vi "Deploy Host Interface.vi"(8 "error in":errorcluster caption="error in (no error)", 10 "resource":string) -> (0 "error out":errorcluster, 2 "resource out":string, 3 "lia host interface":refnum<class "LIA Host Interface.lvclass">)   [LabVIEW 2018, in "Lock-In Amplifier Example Shared.lvlib"]
uses:
  Lock-In Amplifier Example Shared.lvlib
  interface/Interface/LIA Host Interface.lvclass
  interface/Interface RT/LIA Host Interface RT.lvclass
  C:/Users/jfernand/Repositories/Lock-In-Amplifier/Shared/lib/interface/Interface/LIA Host Interface.lvclass
  interface/Interface FPGA/LIA Host Interface FPGA.lvclass
  <vilib>/nisyscfg/nisyscfg.lvlib
  <resource>/objmgr/niflexrioatomicsae.rc
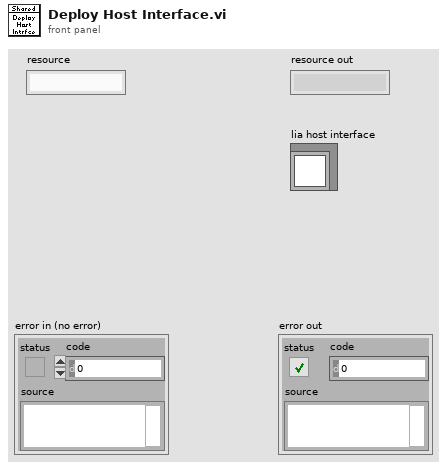
[diagram p1: front panel]
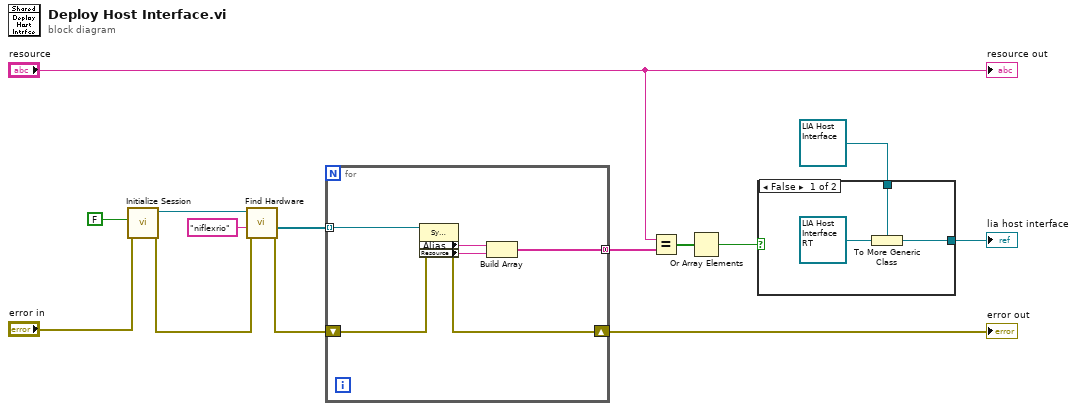
[diagram p0: block diagram]
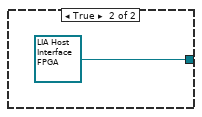
[diagram p2: hidden frame]
diagram:
  n1 = call <vilib>:"Initialize Session.vi"("error in (no error)"="error in", "Force Property Refresh (T)"=FALSE) -> ("error out"=w10:errorcluster, "Session out"=w14:refnum<k21>)  [unwired: 8 in]
  n2 = call <vilib>:"Find Hardware.vi"("error in (no error)"=w10, "Experts"="niflexrio", "Session in"=w14) -> ("error out"=w9:errorcluster, "Resources out"=w11:refnum<k20>[])  [unwired: 5 in, 2 out]
  n3 = for {
    tunnel: w11 -> [w20] mode=indexing
    shift-right: [w18] -> w6
    shift-left: w9 -> [w19]
    tunnel: [w15] -> w8 mode=concatenating
    n4 = property class="System Hardware"(reference=w20, error in=w19) -> (error out=w18:errorcluster, "Alias"=w17:string, "Resource"=w16:string)  [unwired: 1 out]
    n5 = Build Array(w17, w16) -> (w15:string[])
  }
  "error out" <- w6
  n6 = Equal?(x="resource", y=w8) -> (x = y?=w5:bool[])
  n7 = Or Array Elements(Boolean array=w5) -> (logical OR=w4:bool)
  n8 = case shown="False" w4 {
    tunnel: [w22 refnum<class "LIA Host Interface FPGA.lvclass"> refnum ("lia host")] -> w2
    tunnel: refnum<class "LIA Host Interface.lvclass"> refnum ("lia host") -> [w21 _]
    frame False {
      n9 = To More Generic Class(target class=w21, reference=refnum<class "LIA Host Interface RT.lvclass"> refnum ("lia interface rt")) -> (generic class reference=w22:refnum<class "LIA Host Interface.lvclass">)
    }
    frame True {
    }
  }
  "lia host interface" <- w2
  "resource out" <- "resource"
